vi "WildBugChilGru_V0.189.vi"() -> ()   [LabVIEW 2014]
uses:
  <vilib>/Utility/miscctls.llb/LVPointTypeDef.ctl
  <vilib>/Analysis/NI_AALBase.lvlib
  <vilib>/gmath/NI_Gmath.lvlib
  <vilib>/Analysis/NI_AALPro.lvlib
  <vilib>/Utility/NIReport.llb/NI_report.lvclass
  <vilib>/Utility/NIReport.llb/Append Report Text (str wrap).vi
  <vilib>/Instr/_visa.llb/VISA Configure Serial Port (Instr).vi
  <vilib>/Analysis/3filter.llb/IIR Filter (DBL).vi
  <vilib>/Utility/xml.llb/Read From XML File(string).vi
  <vilib>/Utility/xml.llb/Write to XML File(string).vi
panel:
  in  "Registerkarte 2":T1(tab)
  in  "Gleitender Mittelwert":u8=35
  in  "Differenzenquotient":u8=12
  in  "Polynom":u8=15
  in  "n vom Gas [1/min]":dbl=5000.0
  in  "Zündung [Imp/U]":u8=5
  in  "Übersetzung ermitteln aus":T2(ring)
  in  "Getriebe [1:]":dbl=5.343
  in  "Reifenumfang [m]":dbl=1.222
  in  "Dauer [s]":dbl=5.0
  in  "nKuWe/nRolle":dbl=10.0
  in  "Rolle [Inkr/U]":u16=10
  in  "Rollenumfang [m]":dbl=0.613
  in  "Rollenträgheit [kgm²]":dbl=0.402
  in  "Lufttemperatur [°C]":dbl=20.0
  in  "Luftfeuchtigkeit [%]":dbl=50.0
  in  "Luftdruck [mbar]":dbl=1013.0
  in  "Messung":bool
  in  "Ende":bool
  out "Datenspeicher":T3
  out "COM-Fehlerrate":string="0 / 0,0%"
  in  "Konfiguration:":bool
  in  "Speichern":bool
  in  "Drucken":bool
  out "Pmax":string="0,0 PS"
  out "Ergebnis":string="0,0 PS bei 0 1/min   |   0,0 Nm bei 0 1/min   |   vmax: 2147483647 km/h\nDIN 70020 k =1,000 (20 °C, 50 %, 1013 mbar)\n20.11.2016 20:05 "
  in  "Fahrzeugdaten":string="Hier die Fahrzeugdaten eingeben"
  out "XY-Graph":cluster{dbl[], dbl[]}[](graph)
  out "Untersetzung\nermittelt":bool
  out "Untersetzung":dbl format="%#.2f"
  in  "Start [F1]":bool
  out "Füllstand Lesepuffer":u64(slide) scale=1.0..100.0
  out "Hinterrad\n[km/h]":dbl(knob) scale=0.0..150.0
  out "Welle\n[1/min]":cluster{dbl, dbl}(knob) scale=0.0..12000.0
  out "Lesepuffer":string="\n"
  in  "Serielle Schnittstelle":refnum<visa-resource-name>="COM6"
  out "Untersetzung-Graph":dbl(graph)=2.6802446808510636 caption="Untersetzung"
  # "1. n konstant halten\n2. START\n3. n weiter halten\n4. bei GO: Vollgas\n5. vom Gas gehen"
  # "Go"
  # "Zündung\nRolle"
  # "Untersetzung aus:"
  # "Lesen <> Messen"
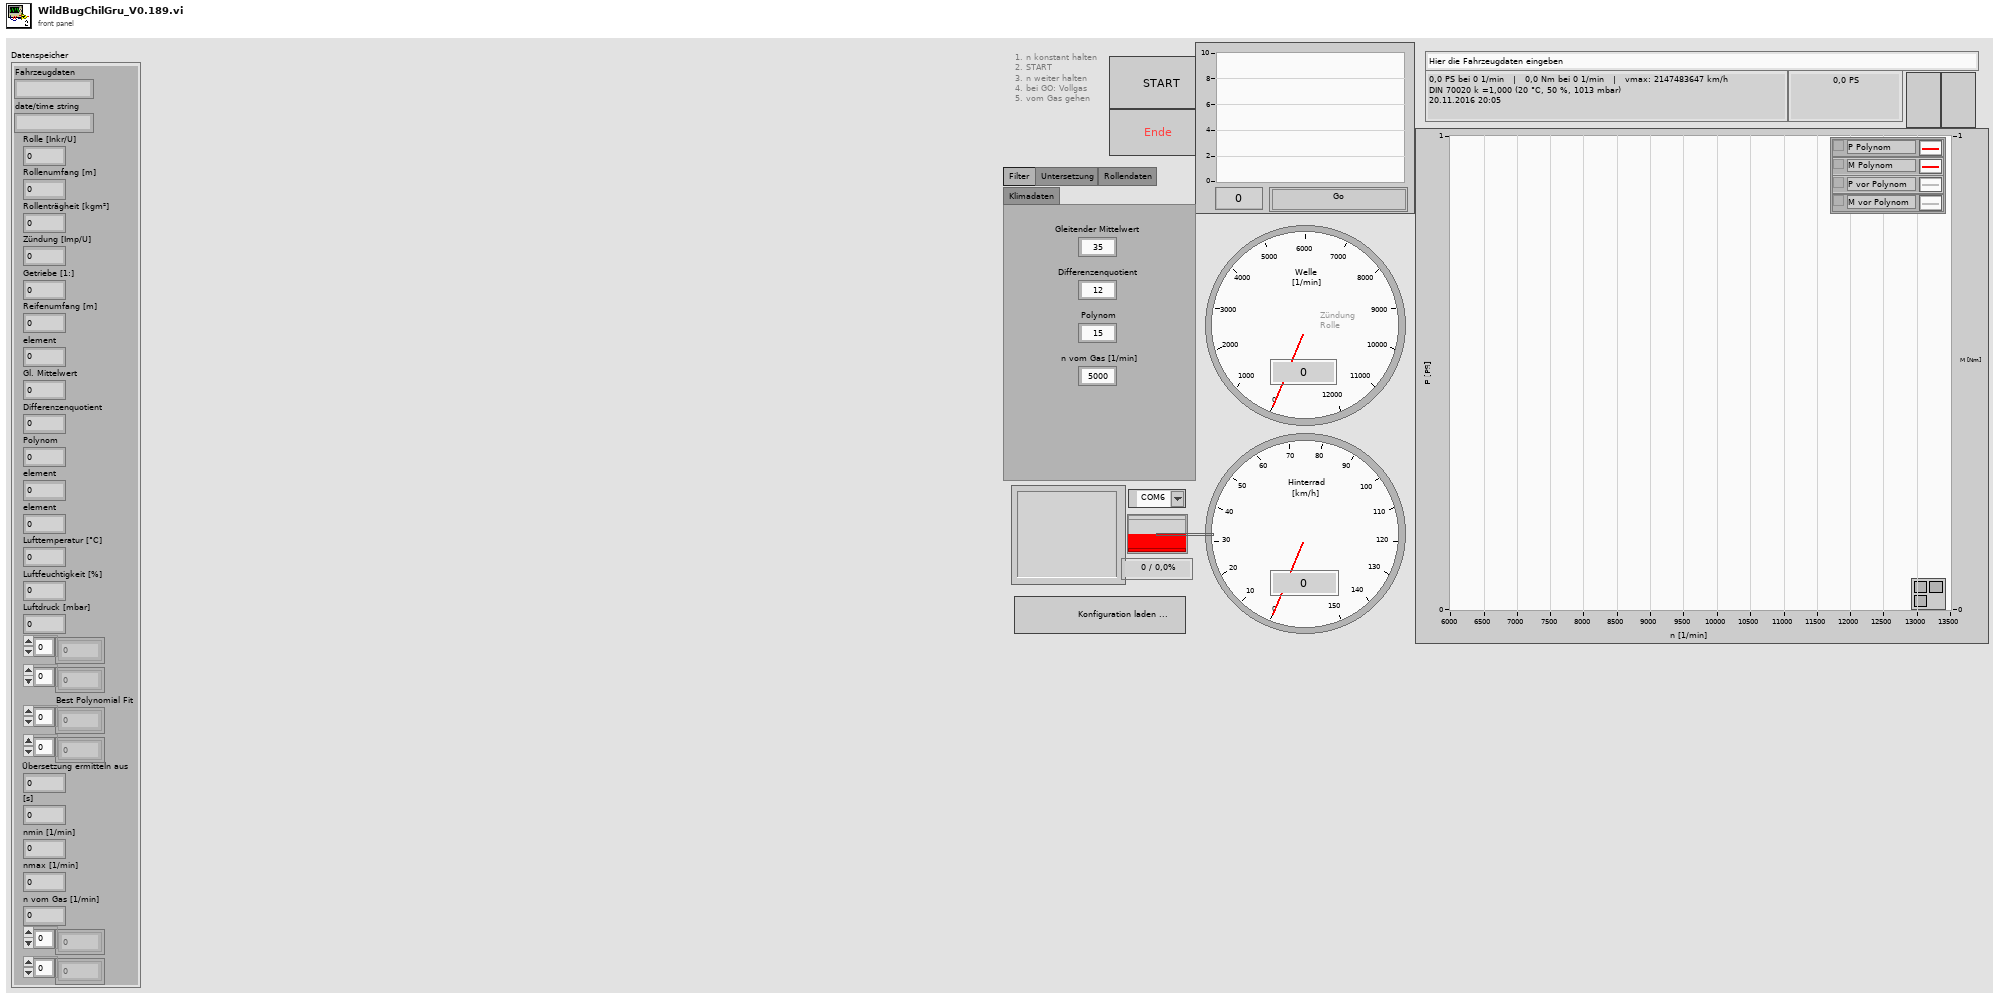
[diagram p1: front panel]
types:
  T1 = enum32{"Filter", "Untersetzung", "Rollendaten", "Klimadaten"}
  T2 = enum8{"Zündsignal", "Getriebe & Reifen", "nKuWe / nRolle"}
  T3 = cluster{"Fahrzeugdaten":string, "date/time string":string, "Rolle [Inkr/U]":u16, "Rollenumfang [m]":dbl, "Rollenträgheit [kgm²]":dbl, "Zündung [Imp/U]":u8, "Getriebe [1:]":dbl, "Reifenumfang [m] ":dbl, "element":dbl, "Gl. Mittelwert":u8, "Differenzenquotient":u8, "Polynom":u8, "element":dbl, "element":dbl, "Lufttemperatur [°C]":dbl, "Luftfeuchtigkeit [%]":dbl, "Luftdruck [mbar]":dbl, dbl[], dbl[], "Best Polynomial Fit":dbl[], dbl[], "Übersetzung ermitteln aus":u8, "[s]":dbl, "nmin [1/min]":dbl, "nmax [1/min]":dbl, "n vom Gas [1/min]":dbl, dbl[], i32[]}
  T4 = enum16{"Kleinste Quadrate", "Kleinestes absolutes Reiduum", "Biquadrat"}
  T5 = enum8{"Enabled", "Disabled", "Disabled and Grayed Out"}
  T6 = cluster{"Fahrzeugdaten":string, "date/time string":string, "Rolle [Inkr/U]":u16, "Rollenumfang [m]":dbl, "Rollenträgheit [kgm²]":dbl, "Zündung [Imp/U]":u8, "Getriebe [1:]":dbl, "Reifenumfang [m] ":dbl, "mean value":dbl, "Gleitender Mittelwert":u8, "Differenzenquotient":u8, "Polynom":u8, dbl, "element":dbl, "Lufttemperatur [°C]":dbl, "Luftfeuchtigkeit [%]":dbl, "Luftdruck [mbar]":dbl, dbl[], dbl[], "Best Polynomial Fit":dbl[], dbl[], "Übersetzung ermitteln aus":enum8{"Zündsignal", "Getriebe & Reifen", "nKuWe / nRolle"}, "Dauer [s]":dbl, dbl, dbl, "n vom Gas [1/min]":dbl, dbl[], i32[]}
  T7 = typedef "LVPointTypeDef.ctl" = cluster{"Horizontal":i16, "Vertical":i16}
  T8 = cluster{string, string, u16, dbl, dbl, u8, dbl, dbl, dbl, u8, u8, u8, dbl, dbl, dbl, dbl, dbl, dbl[], dbl[], dbl[], dbl[], i32, dbl, dbl, dbl, dbl, dbl[], i32[]}
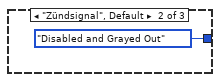
[diagram p2: hidden frame]
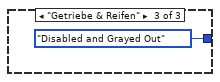
[diagram p3: hidden frame]
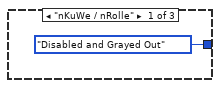
[diagram p4: hidden frame]
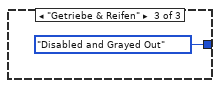
[diagram p5: hidden frame]
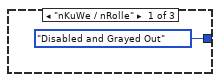
[diagram p6: hidden frame]
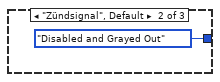
[diagram p7: hidden frame]
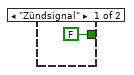
[diagram p10: hidden frame]
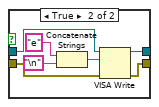
[diagram p12: hidden frame]
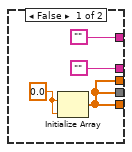
[diagram p14: hidden frame]
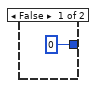
[diagram p15: hidden frame]
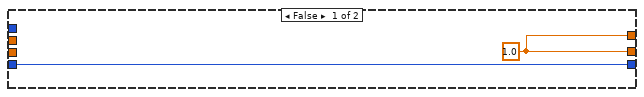
[diagram p17: hidden frame]
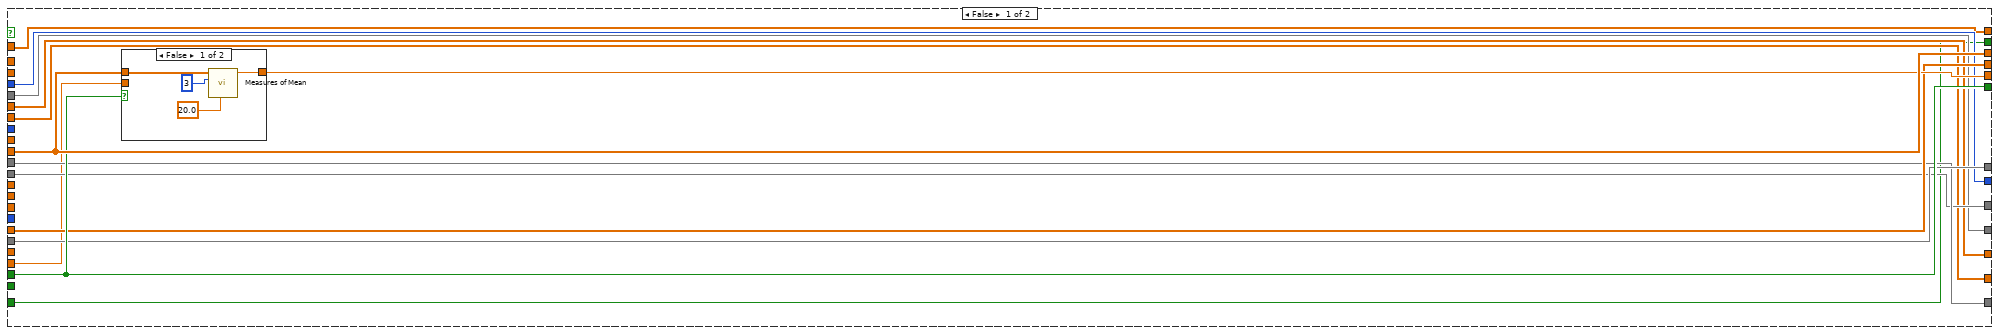
[diagram p18: hidden frame]
diagram:
  n1 = while {
    stop <- w1 stop-if-true
    n2 = event shown="[0] \"Start [F1]\": Wertänderung" {
      selector: _ -> [_ _]
      dyn-events: _ -> [_ _]
      timeout: _ -> [_ _]
      tunnel: [_ TRUE] -> w1
      event "Start [F1]": Value Change {
        n3 = event-data() -> ("NewVal"=w2:bool)  [unwired: 1 in, 5 out]
        n4 = case shown="True" w2 {
          frame False {
          }
          frame True {
            n5 = flat-sequence {
              tunnel: [w132] -> w117
              tunnel: [w131] -> w116
              tunnel: ["Messung"] -> w115
              tunnel: w117 -> [w145]
              tunnel: w116 -> [w144]
              tunnel: [0] -> w114
              tunnel: [1.0 ("element")] -> w113
              tunnel: [FALSE] -> w112
              tunnel: [w157] -> w111
              tunnel: [0] -> w110
              tunnel: [w155] -> w109
              tunnel: [-5] -> w108
              tunnel: [w153] -> w107
              tunnel: [w151] -> w106
              tunnel: [w150] -> w105
              tunnel: [0.0] -> w104
              tunnel: [w145] -> w103
              tunnel: [w144] -> w102
              tunnel: w115 -> [w143]
              tunnel: [w143] -> w101
              tunnel: w114 -> [w182]
              tunnel: [w182] -> w100
              tunnel: w113 -> [w181]
              tunnel: [w181] -> w99
              tunnel: w112 -> [w180]
              tunnel: [w180] -> w98
              tunnel: w111 -> [w179]
              tunnel: [w179] -> w97
              tunnel: w110 -> [w178]
              tunnel: [w178] -> w96
              tunnel: w109 -> [w177]
              tunnel: [w177] -> w95
              tunnel: w108 -> [w176]
              tunnel: [w176] -> w94
              tunnel: w107 -> [w175]
              tunnel: [w175] -> w93
              tunnel: w106 -> [w174]
              tunnel: [w174] -> w92
              tunnel: w105 -> [w173]
              tunnel: [w173] -> w91
              tunnel: w104 -> [w172]
              tunnel: [w172] -> w90
              tunnel: w103 -> [w171]
              tunnel: [w168] -> w89
              tunnel: w102 -> [w170]
              tunnel: [w169] -> w88
              tunnel: [w167] -> w87
              tunnel: w101 -> [w167]
              tunnel: w100 -> [w206]
              tunnel: [w206] -> w86
              tunnel: w99 -> [w205]
              tunnel: [w205] -> w85
              tunnel: w98 -> [w204]
              tunnel: [w204] -> w84
              tunnel: w97 -> [w203]
              tunnel: [w203] -> w83
              tunnel: w96 -> [w202]
              tunnel: [w202] -> w82
              tunnel: w95 -> [w201]
              tunnel: [w201] -> w81
              tunnel: w94 -> [w200]
              tunnel: [w200] -> w80
              tunnel: w93 -> [w199]
              tunnel: [w199] -> w79
              tunnel: w92 -> [w198]
              tunnel: [w198] -> w78
              tunnel: w91 -> [w197]
              tunnel: [w197] -> w77
              tunnel: w90 -> [w196]
              tunnel: [w196] -> w76
              tunnel: w89 -> [w195]
              tunnel: [w195] -> w75
              tunnel: w88 -> [w194]
              tunnel: [w194] -> w74
              tunnel: w87 -> [w192]
              tunnel: [w192] -> w73
              tunnel: w86 -> [w222]
              tunnel: [w222] -> w72
              tunnel: w85 -> [w221]
              tunnel: [w221] -> w71
              tunnel: w84 -> [w220]
              tunnel: [w220] -> w70
              tunnel: w83 -> [w219]
              tunnel: [w219] -> w69
              tunnel: w82 -> [w218]
              tunnel: [w218] -> w68
              tunnel: w81 -> [w217]
              tunnel: [w217] -> w67
              tunnel: w80 -> [w216]
              tunnel: [w216] -> w66
              tunnel: w79 -> [w215]
              tunnel: [w215] -> w65
              tunnel: w78 -> [w214]
              tunnel: [w214] -> w64
              tunnel: w77 -> [w213]
              tunnel: [w213] -> w63
              tunnel: w76 -> [w212]
              tunnel: [w212] -> w62
              tunnel: w75 -> [w211]
              tunnel: [w210] -> w61
              tunnel: w74 -> [w208]
              tunnel: [w209] -> w60
              tunnel: w73 -> [w207]
              tunnel: w72 -> [w298]
              tunnel: w71 -> [w297]
              tunnel: w70 -> [w296]
              tunnel: w69 -> [w295]
              tunnel: w68 -> [w294]
              tunnel: w67 -> [w293]
              tunnel: w66 -> [w292]
              tunnel: w65 -> [w291]
              tunnel: w64 -> [w290]
              tunnel: w63 -> [w289]
              tunnel: w62 -> [w288]
              tunnel: w61 -> [w253]
              tunnel: [w298] -> w59
              tunnel: [w297] -> w58
              tunnel: [w296] -> w57
              tunnel: [w295] -> w56
              tunnel: [w294] -> w55
              tunnel: [w293] -> w54
              tunnel: [w292] -> w53
              tunnel: [w291] -> w52
              tunnel: [w290] -> w51
              tunnel: [w289] -> w50
              tunnel: [w288] -> w49
              tunnel: [w253] -> w48
              tunnel: [w252] -> w47
              tunnel: [w287] -> w46
              tunnel: [w286] -> w45
              tunnel: [w285] -> w44
              tunnel: ["Gleitender Mittelwert"] -> w43
              tunnel: w60 -> [w252]
              tunnel: [w306] -> w9
              tunnel: [w307] -> w10
              tunnel: [w308] -> w11
              tunnel: [w309] -> w12
              tunnel: [w300] -> w7
              tunnel: [w299] -> w8
              tunnel: [w310] -> w13
              tunnel: [w311] -> w14
              tunnel: [w312] -> w16
              tunnel: [w313] -> w18
              tunnel: [w314] -> w19
              tunnel: [w315] -> w20
              tunnel: [w316] -> w37
              tunnel: [w317] -> w39
              tunnel: [w318] -> w40
              tunnel: [w319] -> w41
              tunnel: [w320] -> w42
              tunnel: w59 -> [w320]
              tunnel: w58 -> [w319]
              tunnel: w57 -> [w318]
              tunnel: w56 -> [w317]
              tunnel: w55 -> [w316]
              tunnel: w54 -> [w315]
              tunnel: w53 -> [w314]
              tunnel: w52 -> [w313]
              tunnel: w51 -> [w312]
              tunnel: w50 -> [w311]
              tunnel: w49 -> [w310]
              tunnel: w48 -> [w302]
              tunnel: w47 -> [w301]
              tunnel: w46 -> [w309]
              tunnel: w45 -> [w308]
              tunnel: w44 -> [w307]
              tunnel: w43 -> [w306]
              frame #0 {
                w137 = u16 0 items=["None", "XON/XOFF", "RTS/CTS", "XON/XOFF & RTS/CTS", "DTR/DSR", "XON/XOFF & DTR/DSR"] ("flow control (0:none)")
                w138 = u16 10 items=["1.0"=10, "1.5"=15, "2.0"=20] ("stop bits (10: 1 bit)")
                w130 = FALSE  # Enable Termination Char (T)
                w133 = u32 10000  # timeout (10sec)
                n6 = call-poly "VISA Configure Serial Port"("VISA resource name"="Serielle Schnittstelle", "timeout (10sec)"=w133, "Enable Termination\nChar (T)"=w130, "baud rate (9600)"=u32 250000 ("baudrate (250000)"), "data bits (8)"=u16 8, "parity (0:none)"=enum16{"None", "Odd", "Even", "Mark", "Space"}."None", "stop bits (10: 1 bit)"=w138, "flow control (0:none)"=w137) -> ("VISA resource name out"=w135:refnum<visa-resource-name>, "error out"=w134:errorcluster)  [unwired: 6 in]
                n7 = VISA Clear(VISA resource name=w135, error in (no error)=w134) -> (VISA resource name out=w132:refnum<visa-resource-name>, error out=w131:errorcluster)
              }
              frame #1 {
                w146 = T5."Disabled and Grayed Out" ("Deaktiviert")
                w149 = 0.0  # Graphen löschen
                w152 = 0
                w158 = 0.0
                w150 = ""
                n8 = case shown="True" w143 {
                  frame False {
                  }
                  frame True {
                    n9 = Wait (ms)(milliseconds to wait=u32 2000 ("Zu wartende ms")) -> ()  [unwired: 1 out]
                  }
                }
                n10 = local read "Übersetzung ermitteln aus"() -> (w142:T2)
                n11 = Build Array(w149) -> (w148:dbl[])
                n12 = local write "Pmax"(w150) -> ()
                n13 = property on="Drucken" class="Bool. (strikt)"("DisabledEnum"=w146) -> ()  [unwired: 2 in, 2 out]
                n14 = property on="Übersetzung ermitteln aus" class="Enum (strikt)"("DisabledEnum"=w146) -> ()  [unwired: 2 in, 2 out]
                n15 = property on="Konfiguration:" class="Bool. (strikt)"("DisabledEnum"=w146) -> ()  [unwired: 2 in, 2 out]
                n16 = property on="Ende" class="Bool. (strikt)"("DisabledEnum"=w146) -> ()  [unwired: 2 in, 2 out]
                n17 = property on="Speichern" class="Bool. (strikt)"("DisabledEnum"=w146) -> ()  [unwired: 2 in, 2 out]
                n18 = property on="Untersetzung-Graph" class="SVDiagr (strikt)"("History Data"=w148) -> ()  [unwired: 2 in, 2 out]
                n19 = local write "COM-Fehlerrate"(w150) -> ()
                n20 = local write "Ergebnis"(w150) -> ()
                n21 = case shown="\"Getriebe & Reifen\", Standard" w142 {
                  tunnel: [FALSE TRUE] -> w155
                  frame "Zündsignal" {
                  }
                  frame "Getriebe & Reifen", Default {
                  }
                }
                n22 = Initialize Array(0.0 ("y"), 0) -> (w153:dbl[])
                n23 = Initialize Array(w152, w152) -> (w151:i32[])
                n24 = Initialize Array(w158, w158) -> (w157:dbl[])
              }
              frame #2 {
                n25 = case shown="False" w167 {
                  tunnel: w171 -> [w184 w188]
                  tunnel: w170 -> [w183 w187]
                  tunnel: [w183 w186] -> w169
                  tunnel: [w184 w185] -> w168
                  frame False {
                  }
                  frame True {
                    n26 = Concatenate Strings("e" ("String"), "\n") -> (w191:string)
                    n27 = VISA Write(VISA resource name=w188, write buffer=w191, error in (no error)=w187) -> (VISA resource name out=w185:refnum<visa-resource-name>, error out=w186:errorcluster)  [unwired: 1 out]
                  }
                }
              }
              frame #3 {
                n28 = Wait (ms)(milliseconds to wait=u32 500 ("Zu wartende ms")) -> ()  [unwired: 1 out]
              }
              frame #4 {
                n29 = case shown="True" w207 {
                  tunnel: w211 -> [w224 w247]
                  tunnel: [w224 w246] -> w210
                  tunnel: [w223 w245] -> w209
                  tunnel: w208 -> [w223 w244]
                  frame False {
                  }
                  frame True {
                    n30 = property class="Instr"(reference=w247, error in=w244) -> (reference out=w250:refnum<visa-resource-name>, error out=w249:errorcluster, "Serial Settings:Number of Bytes at Serial Port"=w248:u32)
                    n31 = VISA Read(VISA resource name=w250, byte count=w248, error in (no error)=w249) -> (VISA resource name out=w246:refnum<visa-resource-name>, read buffer=w235:string, error out=w245:errorcluster)  [unwired: 1 out]
                    n32 = Search and Replace String(replace all?=TRUE ("Alle ersetzen? (F)"), input string=w235, search string="." ("Such-String"), replace string="," ("Ersetzungs-String (\"\")")) -> (result string=w234:string)  [unwired: 4 in, 3 out]
                    n33 = String Subset(string=w234, offset (0)=1 ("Offset (0)"), length (rest)=4 ("Länge (Rest)")) -> (substring=w233:string)
                    n34 = String Subset(string=w234, offset (0)=6 ("Offset (0)"), length (rest)=6 ("Länge (Rest)")) -> (substring=w231:string)
                    n35 = String Subset(string=w234, offset (0)=13 ("Offset (0)"), length (rest)=4 ("Länge (Rest)")) -> (substring=w230:string)
                    n36 = Fract/Exp String To Number(string=w233) -> (number=w232:dbl)  [unwired: 3 in, 1 out]
                    n37 = Fract/Exp String To Number(string=w231) -> (number=w227:dbl)  [unwired: 3 in, 1 out]
                    n38 = local write "Lufttemperatur [°C]"(w232) -> ()
                    n39 = Fract/Exp String To Number(string=w230) -> (number=w229:dbl)  [unwired: 3 in, 1 out]
                    n40 = Divide(x=w227, y=100.0 ("x")) -> (x/y=w228:dbl)
                    n41 = local write "Luftdruck [mbar]"(w228) -> ()
                    n42 = local write "Luftfeuchtigkeit [%]"(w229) -> ()
                  }
                }
              }
              frame #5 {
                n43 = Wait (ms)(milliseconds to wait=u32 2000 ("Zu wartende ms")) -> ()  [unwired: 1 out]
                n44 = Add(x="Lufttemperatur [°C]", y=273.15) -> (x+y=w268:dbl)
                n45 = Divide ("M_Welle [Nm]")(x=300.0, y=w268) -> (x/y=w271:dbl)
                n46 = Multiply(x="Luftfeuchtigkeit [%]", y=0.01) -> (x*y=w282:dbl)
                n47 = Divide ("M_Welle [Nm]")(x=w268, y=293.15) -> (x/y=w266:dbl)
                n48 = Multiply(x=w282, y=240800000000.0) -> (x*y=w256:dbl)
                n49 = Power Of X(1:w271, 2:5.0) -> (0:w269:dbl)
                n50 = Multiply(x=w256, y=w269) -> (x*y=w276:dbl)
                n51 = Multiply(x=w271, y=-22.644) -> (x*y=w277:dbl)
                n52 = Power Of X(1:w266, 2:0.5) -> (0:w263:dbl)
                n53 = Exponential(1:w277) -> (0:w275:dbl)
                n54 = Multiply(x=w276, y=w275) -> (x*y=w274:dbl)
                n55 = Subtract "p_Trocken [mbar]"(x="Luftdruck [mbar]", y=w274) -> (x-y=w272:dbl)
                n56 = Divide ("M_Welle [Nm]")(x=1013.0, y=w272) -> (x/y=w264:dbl)
                n57 = Multiply "Korrekturfaktor DIN 70020"(x=w264, y=w263) -> (x*y=w287:dbl)
                n58 = Divide(x="Gleitender Mittelwert", y=2) -> (x/y=w260:dbl)
                n59 = Round Toward -Infinity(1:w260) -> (0:w259:dbl)
                n60 = call <vilib>:"Smoothing Filter Coefficients.vi"("shape"=1, "half-width"=w259, "type"=0) -> ("forward coefficients"=w285:dbl[], "reverse coefficients"=w286:dbl[])  [unwired: 6 in, 1 out]
              }
              frame #6 {
                n61 = Concatenate Strings("m" ("String"), "\n") -> (w305:string)
                n62 = VISA Write(VISA resource name=w302, write buffer=w305, error in (no error)=w301) -> (VISA resource name out=w299:refnum<visa-resource-name>, error out=w300:errorcluster)  [unwired: 1 out]
              }
            }
            n63 = while {
              tunnel: w8 -> [w449]
              tunnel: w7 -> [w448]
              shift-right: [w521] -> _
              shift-left: w14 -> [w465]
              shift-right: [w516] -> _
              shift-left: w13 -> [w520]
              shift-right: [w515] -> _
              shift-left: w13 -> [w519]
              shift-right: [w469] -> _
              shift-left: w13 -> [w518]
              shift-right: [w497] -> _
              shift-left: w42 -> [w517]
              shift-right: [w457] -> w25
              shift-left: w41 -> [_]
              shift-right: [w475] -> w29
              shift-left: w13 -> [w498]
              shift-right: [w508] -> w27
              shift-left: w13 -> [w471]
              shift-right: [w470] -> _
              shift-left: w18 -> [w512]
              shift-right: [w509] -> _
              shift-left: w40 -> [w486]
              shift-right: [w450] -> _
              shift-left: w39 -> [_]
              shift-right: [w456] -> _
              shift-left: w39 -> [_]
              shift-right: [w507] -> w28
              shift-left: w39 -> [w505]
              shift-right: [w506] -> _
              shift-left: w39 -> [w504]
              shift-right: [w492] -> w36
              shift-left: w18 -> [w503]
              shift-right: [w496] -> _
              shift-left: w18 -> [w501]
              shift-right: [w495] -> w32
              shift-left: w18 -> [w502]
              shift-right: [w494] -> w35
              shift-left: w18 -> [w500]
              shift-right: [w493] -> w34
              shift-left: w18 -> [w499]
              tunnel: [w491] -> w38
              shift-right: [w487] -> w33
              shift-left: w37 -> [w489]
              tunnel: [w490] -> w3
              tunnel: ["n vom Gas [1/min]"] -> w31
              tunnel: ["Rollenumfang [m]"] -> w30
              tunnel: ["Rollenumfang [m]"] -> w24
              shift-right: [w482] -> _
              shift-left: w20 -> [w483]
              shift-right: [w476] -> _
              shift-left: w19 -> [w481]
              shift-right: [w477] -> _
              shift-left: w13 -> [w480]
              shift-right: [w478] -> _
              shift-left: w13 -> [w479]
              shift-right: [w474] -> w17
              shift-left: w18 -> [w473]
              shift-right: [w468] -> _
              shift-left: _ -> [w467]
              shift-right: [w472] -> w15
              shift-left: w16 -> [w466]
              tunnel: [w464] -> w4
              tunnel: w12 -> [w457]
              tunnel: w11 -> [w450]
              tunnel: w10 -> [w456]
              tunnel: w9 -> [w455]
              stop <- w491 stop-if-true
              n64 = property class="Instr"(reference=w449, error in=w448) -> (reference out=w460:refnum<visa-resource-name>, error out=w459:errorcluster, "Serial Settings:Number of Bytes at Serial Port"=w462:u32)
              n65 = Greater?(x=w462, y=u32 1 ("min. Bytes")) -> (0:w458:bool)
              n66 = case shown="True" w458 {
                tunnel: w462 -> [_ w523]
                tunnel: [u32 0 ("Bytes at Port") w523] -> w461
                frame False {
                }
                frame True {
                }
              }
              n67 = case shown="1.." w461 {
                selector: w461 -> [_ w769]
                tunnel: [w719 w763] -> w490
                tunnel: [w718 w764] -> w464
                tunnel: [w723 w765] -> w515
                tunnel: [w724 w762] -> w516
                tunnel: w465 -> [w725 w760]
                tunnel: [w725 w758] -> w521
                tunnel: w520 -> [w724 w750]
                tunnel: w519 -> [w723 w749]
                tunnel: [w720 w748] -> w469
                tunnel: w518 -> [w720 w747]
                tunnel: w517 -> [w722 _]
                tunnel: [w722 w730] -> w497
                tunnel: [w721 w736] -> w468
                tunnel: w467 -> [w721 w735]
                tunnel: w460 -> [w718 w727]
                tunnel: w459 -> [w719 w726]
                frame 0, Default {
                  # "No data in from serial port - Nothing to do."
                }
                frame 1.. {
                  # "Hz Drum"
                  n68 = VISA Read(VISA resource name=w727, byte count=w769, error in (no error)=w726) -> (VISA resource name out=w764:refnum<visa-resource-name>, read buffer=w761:string, error out=w763:errorcluster)  [unwired: 1 out]
                  n69 = Concatenate Strings(w760, w761) -> (w732:string)
                  "Lesepuffer" <- w732
                  n70 = Spreadsheet String To Array(delimiter (Tab)="\n" ("regular expression"), format string="%s" ("regular expression"), spreadsheet string=w732, array type (2D Dbl)=string[] [] ("Array 2")) -> (array=w741:string[])
                  n71 = Match Pattern(string=w732, regular expression="[\\n]") -> (before substring=w739:string, after substring=w759:string, offset past match=w773:i32)  [unwired: 1 in, 1 out]
                  n72 = Array Size(array=w741) -> (size(s)=w745:i32)
                  n73 = Match Pattern(string=w739, regular expression="[;]") -> (before substring=w737:string, after substring=w738:string, offset past match=w734:i32)  [unwired: 1 in, 1 out]
                  n74 = Subtract "aktuelle Zeilenanzahl"(x=w745, y=1) -> (x-y=w730:i32)
                  n75 = property on="Füllstand Lesepuffer" class="Schieber (strikt)"() -> ("Scale.Maximum"=w729:dbl)  [unwired: 2 in, 2 out]
                  n76 = Match Pattern(string=w738, regular expression="[;]") -> (before substring=w768:string, after substring=w771:string, offset past match=w756:i32)  [unwired: 1 in, 1 out]
                  n77 = Match Pattern(string=w771, regular expression="[;]") -> (before substring=w767:string, after substring=w766:string, offset past match=w754:i32)  [unwired: 1 in, 1 out]
                  n78 = Greater?(x=w730, y=w729) -> (0:w731:bool)
                  n79 = Greater Or Equal To 0?(x=w734) -> (x >= 0?=w733:bool)
                  n80 = Greater Or Equal To 0?(x=w754) -> (x >= 0?=w753:bool)
                  n81 = Greater Or Equal To 0?(x=w756) -> (x >= 0?=w755:bool)
                  n82 = Greater Or Equal To 0?(x=w773) -> (x >= 0?=w757:bool)
                  n83 = Select(t=w730, s=w731, f=w729) -> (s? t:f=w728:dbl)
                  n84 = property on="Füllstand Lesepuffer" class="Schieber (strikt)"("Scale.Maximum"=w728) -> ()  [unwired: 2 in, 2 out]
                  n85 = Build Array(w757, w755, w733, w753) -> (w752:bool[])
                  n86 = And Array Elements(Boolean array=w752) -> (logical AND=w751:bool)
                  n87 = case shown="True" w751 {
                    tunnel: w768 -> [_ w784]
                    tunnel: w767 -> [_ w789]
                    tunnel: w766 -> [_ w788]
                    tunnel: [w777 w787] -> w765
                    tunnel: [w778 w786] -> w762
                    tunnel: w759 -> [_ w785]
                    tunnel: [w779 w785] -> w758
                    tunnel: w732 -> [w779 _]
                    tunnel: w750 -> [w778 _]
                    tunnel: w749 -> [w777 _]
                    tunnel: [w776 w783] -> w748
                    tunnel: w747 -> [w776 _]
                    tunnel: w737 -> [_ w782]
                    tunnel: [w775 w780] -> w736
                    tunnel: w735 -> [w775 _]
                    frame False {
                    }
                    frame True {
                      # "Cyclecounter"
                      # "Hz ComLevel"
                      # "ComLevel\nLevel 10 =   6Hz \nLevel 5 =   12Hz \nLevel 4 =   15Hz\nLevel 3 =   20Hz\nLevel 2 =   33Hz\nLevel 1 =   62Hz"
                      # "Hz Drum"
                      # "Hz Engine"
                      # "t4m"
                      n88 = Fract/Exp String To Number(string=w782) -> (number=w781:dbl)  [unwired: 3 in, 1 out]
                      n89 = Fract/Exp String To Number(string=w788) -> (number=w787:dbl)  [unwired: 3 in, 1 out]
                      n90 = Fract/Exp String To Number(string=w784) -> (number=w783:dbl)  [unwired: 3 in, 1 out]
                      n91 = To Long Integer(number=w781) -> (32bit integer=w780:i32)
                      n92 = Fract/Exp String To Number(string=w789) -> (number=w786:dbl)  [unwired: 3 in, 1 out]
                    }
                  }
                }
              }
              "Füllstand Lesepuffer" <- w497
              n93 = Not Equal?(x=w467, y=w468) -> (x != y?=w451:bool)
              n94 = case shown="True" w451 {
                tunnel: w481 -> [w527 w538]
                tunnel: [w527 w550] -> w476
                tunnel: w480 -> [w526 w549]
                tunnel: [w526 w535] -> w477
                tunnel: w479 -> [w525 w548]
                tunnel: [w525 w536] -> w478
                tunnel: w468 -> [_ w534]
                tunnel: w466 -> [w524 w533]
                tunnel: [w524 w537] -> w472
                frame False {
                }
                frame True {
                  n95 = Build Array (concatenate)(w533, w534) -> (w537:i32[])
                  n96 = Greater Or Equal To 0?(x=w538) -> (x >= 0?=w539:bool)
                  n97 = case shown="True" w539 {
                    tunnel: [w551 w562] -> w535
                    tunnel: [w551 w563] -> w536
                    tunnel: [w552 w554] -> w550
                    tunnel: w549 -> [_ w556]
                    tunnel: w548 -> [_ w564]
                    tunnel: w534 -> [w552 w553]
                    tunnel: w538 -> [_ w554]
                    frame False {
                      w551 = 1.0
                    }
                    frame True {
                      w560 = 65536.0
                      n98 = Add(x=w554, y=w556) -> (x+y=w555:dbl)
                      n99 = Divide(x=w555, y=w560) -> (x/y=w565:dbl)
                      n100 = Increment(x=w564) -> (x+1=w563:dbl)
                      n101 = Round Toward -Infinity(1:w565) -> (0:w561:dbl)
                      n102 = Multiply(x=w561, y=w560) -> (x*y=w559:dbl)
                      n103 = Add(x=w559, y=w553) -> (x+y=w558:dbl)
                      n104 = Increment(x=w558) -> (x+1=w557:dbl)
                      n105 = Subtract(x=w557, y=w554) -> (x-y=w562:dbl)
                    }
                  }
                  n106 = Subtract(x=w535, y=w536) -> (x-y=w530:dbl)
                  n107 = Decrement(x=w530) -> (x-1=w529:dbl)
                  n108 = Max & Min(x=0, y=w529) -> (max(x,y)=w528:dbl)  [unwired: 1 out]
                  n109 = Divide(x=w528, y=w535) -> (x/y=w542:dbl)
                  n110 = Greater Than 0?(x=w528) -> (x > 0?=w532:bool)
                  n111 = Select(t=u32 16711680, s=w532, f=u32 0) -> (s? t:f=w543:u32)
                  n112 = Multiply(x=w542, y=100.0) -> (x*y=w540:dbl)
                  n113 = property on="COM-Fehlerrate" class="Str"("Text.TextColor"=w543) -> ()  [unwired: 2 in, 2 out]
                  n114 = Format Into String(format string="%d / %.1f%%" ("Format-String"), w528, w540) -> (resulting string=→"COM-Fehlerrate":string)  [unwired: 2 in, 1 out]
                }
              }
              n115 = case "Case-Struktur" shown="True" w451 {
                tunnel: w516 -> [w699 w710]
                tunnel: w515 -> [w698 w709]
                tunnel: [w699 w708] -> w514
                tunnel: [w698 w707] -> w513
                tunnel: w469 -> [_ w701]
                tunnel: w498 -> [w697 _]
                tunnel: [w697 w700] -> w475
                tunnel: w471 -> [_ w706]
                tunnel: "Rollenumfang [m]" -> [_ w705]
                frame False {
                }
                frame True {
                  w717 = 60.0 ("y")
                  n116 = Reciprocal "Abtastzeit [s]"(x=w701) -> (1/x=w700:dbl)
                  n117 = Divide "R [1/s]"(x=w709, y="Rolle [Inkr/U]") -> (x/y=w716:dbl)
                  n118 = Multiply "nR [1/min]"(x=w717, y=w716) -> (x*y=w707:dbl)
                  n119 = Divide(x=w710, y="Zündung [Imp/U]") -> (x/y=w713:dbl)
                  n120 = Multiply "nZ gemessen [1/min]"(x=w713, y=w717) -> (x*y=w708:dbl)
                  n121 = Multiply "nZ berechnet [1/min]"(x=w707, y=w706) -> (x*y=w715:dbl)
                  n122 = Multiply "[m/min]"(x=w707, y=w705) -> (x*y=w711:dbl)
                  n123 = Multiply "[km/h]"(x=w711, y=0.06) -> (x*y=→"Hinterrad\n[km/h]":dbl)
                  n124 = Bundle(w708, w715) -> (→"Welle\n[1/min]":cluster{dbl, dbl})  [unwired: 1 in]
                }
              }
              n125 = local read "Übersetzung ermitteln aus"() -> (w452:T2)
              n126 = case shown="True" w451 {
                tunnel: w514 -> [_ w634]
                tunnel: w513 -> [_ w633]
                tunnel: "Rollenumfang [m]" -> [_ w637]
                tunnel: [w577 w603] -> w508
                tunnel: w471 -> [w566 w603]
                tunnel: w452 -> [_ w642]
                tunnel: w486 -> [w578 w641]
                tunnel: w512 -> [w579 w640]
                tunnel: [w578 w594] -> w509
                tunnel: [w579 w639] -> w470
                tunnel: w450 -> [_ w636]
                tunnel: w456 -> [_ w635]
                tunnel: [w576 w589] -> w507
                tunnel: [w575 w587] -> w506
                tunnel: w505 -> [w576 w632]
                tunnel: w504 -> [w575 _]
                tunnel: w455 -> [_ w585]
                tunnel: [w574 w609] -> w492
                tunnel: w503 -> [w574 _]
                tunnel: [w573 w624] -> w496
                tunnel: w501 -> [w573 _]
                tunnel: w498 -> [_ w622]
                tunnel: [w572 w610] -> w495
                tunnel: w502 -> [w572 _]
                tunnel: [w571 w626] -> w494
                tunnel: w500 -> [w571 _]
                tunnel: [w570 w625] -> w493
                tunnel: w499 -> [w570 _]
                tunnel: w457 -> [_ w614]
                tunnel: w489 -> [w569 w608]
                tunnel: "n vom Gas [1/min]" -> [_ w596]
                tunnel: [w569 w607] -> w487
                tunnel: w486 -> [_ w606]
                tunnel: w483 -> [w568 w602]
                tunnel: [w568 w601] -> w482
                tunnel: w475 -> [_ w600]
                tunnel: [w567 w599] -> w474
                tunnel: w473 -> [w567 w598]
                frame False {
                  n127 = case shown="False" w578 {
                    tunnel: w579 -> [w583 _]
                    tunnel: [w582 w584] -> w577
                    tunnel: w566 -> [_ w584]
                    frame False {
                      n128 = call <vilib>:"Measures of Mean.vi"("percent (trim)"=20.0, "type"=3, "x array"=w583) -> ("mean value"=w582:dbl)  [unwired: 7 in, 1 out]
                    }
                    frame True {
                    }
                  }
                }
                frame True {
                  w617 = 0.00135962  # [W] in [PS]
                  w628 = 0.10471975511965978  # 2*Pi/60
                  n129 = Build Array (concatenate) "akt. dT in Array einfügen"(w598, w600) -> (w599:dbl[])
                  n130 = case shown="\"Getriebe & Reifen\"" w642 {
                    tunnel: w634 -> [_ _ w696]
                    tunnel: w633 -> [_ _ w695]
                    tunnel: [w691 "nKuWe/nRolle" w694] -> w638
                    tunnel: w637 -> [w692 _ _]
                    frame "Getriebe & Reifen" {
                      n131 = Divide(x=w692, y="Reifenumfang [m]") -> (x/y=w690:dbl)
                      n132 = Multiply(x=w690, y="Getriebe [1:]") -> (x*y=w691:dbl)
                    }
                    frame "nKuWe / nRolle" {
                    }
                    frame "Zündsignal" {
                      n133 = Divide(x=w696, y=w695) -> (x/y=w694:dbl)
                    }
                  }
                  n134 = Build Array (concatenate) "akt. Rollendrehzahl\nin Array einfügen"(w632, w633) -> (w589:dbl[])
                  n135 = Index Array(array=w589, index=1 ("Index")) -> (element=w592:dbl)
                  n136 = Initialize Array(w592, w585) -> (w591:dbl[])
                  n137 = Insert Into Array(array=w589, index=0 ("Index"), new element=w591) -> (w588:dbl[])
                  n138 = call-poly <vilib>:"IIR Filter.vi"("Forward Coefficients"=w635, "Reverse Coefficients"=w636, "X"=w588) -> ("Filtered X"=w586:dbl[])  [unwired: 1 in, 1 out]
                  n139 = Array Subset(array=w586, index=w585) -> (w587:dbl[])  [unwired: 1 in]
                  n140 = Multiply(x=2.0, y=w622) -> (x*y=w621:dbl)
                  n141 = case shown="False" w641 {
                    selector: w641 -> [_ w687]
                    tunnel: w638 -> [w682 _]
                    tunnel: w640 -> [w684 w686]
                    tunnel: [w679 w687] -> w631
                    tunnel: [w683 w686] -> w639
                    tunnel: w602 -> [w680 w685]
                    tunnel: [w679 w685] -> w601
                    frame False {
                      n142 = Build Array (concatenate)(w684, w682) -> (w683:dbl[])
                      n143 = call "Verstrichene Zeit"("Time Target (s)"="Dauer [s]", "Reset"=w680) -> ("Time has Elapsed"=w679:bool)  [unwired: 10 in, 7 out]
                      "Untersetzung-Graph" <- w682
                    }
                    frame True {
                    }
                  }
                  n144 = Array Size "Array-Größe"(array=w587) -> (size(s)=w629:i32)
                  n145 = Square(x=w603) -> (x^2=w627:dbl)
                  n146 = Multiply(x=w587, y=w603) -> (x*y=w609:dbl[])
                  n147 = Divide(x="Rollenträgheit [kgm²]", y=w627) -> (x/y=w615:dbl)
                  n148 = Greater?(x=w629, y=w585) -> (0:w630:bool)
                  n149 = Multiply(x=w609, y=w628) -> (x*y=w624:dbl[])
                  n150 = Multiply(x=w615, y=w614) -> (x*y=w613:dbl)
                  n151 = And(x=w631, y=w630) -> (x .and. y?=w594:bool)
                  n152 = Array Size "Array-Größe"(array=w624) -> (size(s)=w612:i32)
                  n153 = Decrement(x=w612) -> (x-1=w611:i32)
                  n154 = Select(t=w596, s=w594, f=1000000.0) -> (s? t:f=w597:dbl)
                  n155 = Initialize Array(0.0 ("y"), 0) -> (w618:dbl[])
                  n156 = for {
                    N: w612 -> [_]
                    tunnel: "Differenzenquotient" -> [w654]
                    tunnel: w624 -> [w662]
                    tunnel: w611 -> [w653]
                    tunnel: w621 -> [w663]
                    shift-right: [w659] -> w610
                    shift-left: w618 -> [w660]
                    tunnel: w609 -> [w657] mode=indexing
                    tunnel: w608 -> [w645]
                    tunnel: w597 -> [w656]
                    tunnel: [w646] -> w607
                    tunnel: w606 -> [w643]
                    i -> [w647]
                    stop <- w644 stop-if-true
                    n157 = Subtract(x=w653, y=w654) -> (x-y=w655:i32)
                    n158 = Add(x=w647, y=w654) -> (x+y=w670:i32)
                    n159 = Subtract(x=w647, y=w654) -> (x-y=w676:i32)
                    n160 = Greater Or Equal?(x=w647, y=w654) -> (x >= y?=w650:bool)
                    n161 = Greater?(x=w657, y=w656) -> (0:w658:bool)
                    n162 = Max & Min(x=w653, y=w670) -> (min(x,y)=w671:i32)  [unwired: 1 out]
                    n163 = Max & Min(x=w676, y=0) -> (max(x,y)=w674:i32)  [unwired: 1 out]
                    n164 = Less Or Equal?(x=w647, y=w655) -> (x <= y?=w651:bool)
                    n165 = Subtract(x=w671, y=w647) -> (x-y=w672:i32)
                    n166 = Subtract(x=w647, y=w674) -> (x-y=w673:i32)
                    n167 = Max & Min(x=w673, y=w672) -> (min(x,y)=w664:i32)  [unwired: 1 out]
                    n168 = Multiply(x=w664, y=w663) -> (x*y=w661:dbl)
                    n169 = Add(x=w647, y=w664) -> (x+y=w669:i32)
                    n170 = Subtract(x=w647, y=w664) -> (x-y=w668:i32)
                    n171 = Index Array(array=w662, index=w669) -> (element=w666:dbl)
                    n172 = Index Array(array=w662, index=w668) -> (element=w667:dbl)
                    n173 = Subtract(x=w666, y=w667) -> (x-y=w665:dbl)
                    n174 = Divide(x=w665, y=w661) -> (x/y=w652:dbl)
                    n175 = Less Or Equal To 0?(x=w645) -> (x <= 0?=w648:bool)
                    n176 = Less Than 0?(x=w652) -> (x < 0?=w649:bool)
                    n177 = Build Array (concatenate)(w660, w652) -> (w659:dbl[])
                    n178 = Compound Arithmetic op=AND(w649, w658, w648, w650, w651, w643) -> (w644:bool)
                    n179 = case shown="True" w644 {
                      tunnel: w647 -> [_ w678]
                      tunnel: [w677 w678] -> w646
                      tunnel: w645 -> [w677 _]
                      frame False {
                      }
                      frame True {
                      }
                    }
                  }
                  n180 = Multiply(x=w610, y=w613) -> (x*y=w626:dbl[])
                  n181 = Multiply(x=w624, y=w626) -> (x*y=w616:dbl[])
                  n182 = Multiply(x=w617, y=w616) -> (x*y=w625:dbl[])
                }
              }
              "Untersetzung\nermittelt" <- w509
              n183 = local read "Start [F1]"() -> (w454:bool)
              n184 = Not(x=w454) -> (.not. x?=w453:bool)
              n185 = Greater Than 0?(x=w487) -> (x > 0?=w488:bool)
              n186 = Select(t=w508, s=w509, f=0.0) -> (s? t:f=→"Untersetzung":dbl)
              n187 = Or(x=w488, y=w453) -> (x .or. y?=w491:bool)
            }
            n188 = VISA Clear(VISA resource name=w4, error in (no error)=w3) -> (VISA resource name out=w5:refnum<visa-resource-name>, error out=w6:errorcluster)
            n189 = VISA Close(VISA resource name=w5, error in (no error)=w6) -> ()  [unwired: 1 out]
            n190 = case shown="True" w38 {
              tunnel: w36 -> [_ w424]
              tunnel: w35 -> [_ w429]
              tunnel: w34 -> [_ w428]
              tunnel: w33 -> [_ w400]
              tunnel: w32 -> [_ w425]
              tunnel: w31 -> [_ w423]
              tunnel: w30 -> [_ w417]
              tunnel: w25 -> [_ w403]
              tunnel: ["" w402] -> w26
              tunnel: w27 -> [_ w401]
              tunnel: ["" w399] -> _
              tunnel: [w363 w376] -> w23
              tunnel: [w363 w375] -> w22
              tunnel: [w363 w374] -> w21
              frame False {
                w364 = 0.0
                n191 = Initialize Array(w364, w364) -> (w363:dbl[])
              }
              frame True {
                w388 = 735.498  # PS in W
                w394 = 0.10471975511965978  # w = (2 * Pi / 60) * n
                w398 = 0
                n192 = Array Subset "P"(array=w428, length=w400) -> (w420:dbl[])  [unwired: 1 in]
                n193 = Array Subset "M"(array=w429, length=w400) -> (w421:dbl[])  [unwired: 1 in]
                n194 = Array Subset "alpha"(array=w425, length=w400) -> (w426:dbl[])  [unwired: 1 in]
                n195 = Array Subset "n"(array=w424, length=w400) -> (w422:dbl[])  [unwired: 1 in]
                n196 = property on="Pmax" class="Str"("Text.FontSize"=48) -> ()  [unwired: 2 in, 2 out]
                n197 = property on="Ergebnis" class="Str"("Text.FontSize"=18) -> ()  [unwired: 2 in, 2 out]
                n198 = Array Size(array=w426) -> (size(s)=w427:i32)
                n199 = for {
                  N: w427 -> [w447]
                  tunnel: w425 -> [w444]
                  tunnel: w424 -> [w441]
                  tunnel: w423 -> [w438]
                  tunnel: [w436] -> w396
                  i -> [w442]
                  stop <- w437 stop-if-true
                  n200 = Decrement(x=w447) -> (x-1=w446:i32)
                  n201 = Subtract(x=w446, y=w442) -> (x-y=w436:i32)
                  n202 = Index Array(array=w444, index=w436) -> (element=w445:dbl)
                  n203 = Index Array(array=w441, index=w436) -> (element=w440:dbl)
                  n204 = Less?(x=w440, y=w438) -> (x < y?=w439:bool)
                  n205 = Less Or Equal To 0?(x=w445) -> (x <= 0?=w443:bool)
                  n206 = And(x=w443, y=w439) -> (x .and. y?=w437:bool)
                }
                n207 = Increment(x=w396) -> (x+1=w395:i32)
                n208 = Array Subset "P"(array=w420, index=w395) -> (w397:dbl[])  [unwired: 1 in]
                n209 = Array Subset "M"(array=w421, index=w395) -> (w393:dbl[])  [unwired: 1 in]
                n210 = Array Subset "n"(array=w422, index=w395) -> (w376:dbl[])  [unwired: 1 in]
                n211 = local write "Polynom"("Polynom") -> ()
                n212 = Array Max & Min "nmax [1/min]"(array=w376) -> (max value=w419:dbl)  [unwired: 3 out]
                n213 = Bundle(w376, w397) -> (w380:cluster{dbl[], dbl[]})  [unwired: 1 in]
                n214 = Bundle(w376, w393) -> (w381:cluster{dbl[], dbl[]})  [unwired: 1 in]
                n215 = Multiply(x=w376, y=w394) -> (x*y=w390:dbl[])
                n216 = Array Size(array=w376) -> (size(s)=w373:i32)
                n217 = call <vilib>:"General Polynomial Fit.vi"("Y"=w393, "polynomial order"="Polynom", "X"=w376, "method"=T4."Biquadrat" ("Methode"), "algorithm"=3) -> ("Best Polynomial Fit"=w375:dbl[])  [unwired: 7 in, 3 out]
                n218 = Bundle(w376, "Best Polynomial Fit"=w375) -> (w382:cluster{dbl[], "Best Polynomial Fit":dbl[]})  [unwired: 1 in]
                n219 = Multiply(x=w375, y=w390) -> (x*y=w389:dbl[])
                n220 = Multiply(x=w373, y=0.1) -> (x*y=w367:dbl)
                n221 = Multiply(x=w373, y=0.8) -> (x*y=w384:dbl)
                n222 = Array Subset "MPoly ohne die ersten\nund letzten paar %"(array=w375, index=w367, length=w384) -> (w378:dbl[])
                n223 = Array Subset "n ohne die ersten \nund letzten paar %"(array=w376, index=w367, length=w384) -> ()  [unwired: 1 out]
                n224 = Divide(x=w419, y=w401) -> (x/y=w418:dbl)
                n225 = Divide(x=w389, y=w388) -> (x/y=w374:dbl[])
                n226 = Array Subset "PPoly ohne die ersten\nund letzten paar %"(array=w374, index=w367, length=w384) -> (w379:dbl[])
                n227 = Bundle(w376, w374) -> (w383:cluster{dbl[], dbl[]})  [unwired: 1 in]
                n228 = Compound Arithmetic op=MULTIPLY "vmax"(w418, w417, 0.06) -> (w409:dbl)
                n229 = Array Max & Min "Mmax"(array=w378) -> (max value=w386:dbl, max index (indices)=w369:i32)  [unwired: 2 out]
                n230 = Add(x=w367, y=w369) -> (x+y=w368:dbl)
                n231 = Multiply(x=w386, y=1.8) -> (x*y=w430:dbl)
                n232 = Index Array "n(Mmax)"(array=w376, index=w368) -> (element=w410:dbl)
                n233 = Array Max & Min "Pmax"(array=w379) -> (max value=w387:dbl, max index (indices)=w371:i32)  [unwired: 2 out]
                n234 = Build Array(w383, w382, w380, w381) -> (→"XY-Graph":cluster{dbl[], "Best Polynomial Fit":dbl[]}[])
                n235 = Add(x=w367, y=w371) -> (x+y=w370:dbl)
                n236 = local read "Luftfeuchtigkeit [%]"() -> (w413:dbl)
                n237 = Multiply(x=w387, y=1.2) -> (x*y=w431:dbl)
                n238 = local read "Lufttemperatur [°C]"() -> (w412:dbl)
                n239 = local read "Luftdruck [mbar]"() -> (w414:dbl)
                n240 = property on="XY-Graph" class="XYGraph (strikt)"("ActYScl"=1, "YScale.Maximum"=w430, "YScale.Minimum"=w398) -> ()  [unwired: 2 in, 2 out]
                n241 = property on="XY-Graph" class="XYGraph (strikt)"("ActYScl"=w398, "YScale.Maximum"=w431, "YScale.Minimum"=w398) -> ()  [unwired: 2 in, 2 out]
                n242 = Index Array "n(Pmax)"(array=w376, index=w370) -> (element=w415:dbl)
                n243 = Format Into String(format string="%.1f PS" ("Format-String"), w387) -> (resulting string=→"Pmax":string)  [unwired: 2 in, 1 out]
                n244 = Format Date/Time String(time format string (%c)="%x %H:%M ") -> (date/time string=w402:string)  [unwired: 2 in]
                n245 = Format Into String(format string="%.1f PS bei %d 1/min   |   %.1f Nm bei %d 1/min   |   vmax: %d km/h\\nDIN 70020 k =%.3f (%d \\B0C, %d %%, %d mbar)\\n%s" ("Format-String"), w387, w415, w386, w410, w409, w403, w412, w413, w414, w402) -> (resulting string=w399:string)  [unwired: 2 in, 1 out]
                "Ergebnis" <- w399
              }
            }
            n246 = flat-sequence {
              tunnel: w15 -> [w324]
              tunnel: w17 -> [w325]
              tunnel: w21 -> [w326]
              tunnel: w22 -> [w327]
              tunnel: w23 -> [w328]
              tunnel: w24 -> [w329]
              tunnel: w25 -> [w330]
              tunnel: w26 -> [w331]
              tunnel: w27 -> [w332]
              tunnel: w28 -> [w333]
              tunnel: w29 -> [w334]
              tunnel: [w334] -> w128
              tunnel: [w333] -> w127
              tunnel: [w332] -> w126
              tunnel: [w331] -> w125
              tunnel: [w330] -> w124
              tunnel: [w329] -> w123
              tunnel: [w328] -> w122
              tunnel: [w327] -> w121
              tunnel: [w326] -> w120
              tunnel: [w325] -> w119
              tunnel: [w324] -> w118
              tunnel: w128 -> [w362]
              tunnel: w127 -> [w361]
              tunnel: w126 -> [w360]
              tunnel: w125 -> [w359]
              tunnel: w124 -> [w358]
              tunnel: w123 -> [w357]
              tunnel: w122 -> [w356]
              tunnel: w121 -> [w355]
              tunnel: w120 -> [w354]
              tunnel: w119 -> [w353]
              tunnel: w118 -> [w352]
              frame #0 {
                w322 = FALSE ("Start [F1]")
                w323 = 0  # Aktivieren
                n247 = property on="XY-Graph" class="XYGraph (strikt)"("YScale.ScaleFit"=u8 1 ("X-Achse.Achsenanpassung")) -> ()  [unwired: 2 in, 2 out]
                n248 = property on="Speichern" class="Bool. (strikt)"("DisabledEnum"=w323) -> ()  [unwired: 2 in, 2 out]
                n249 = property on="Übersetzung ermitteln aus" class="Enum (strikt)"("DisabledEnum"=w323) -> ()  [unwired: 2 in, 2 out]
                n250 = property on="Konfiguration:" class="Bool. (strikt)"("DisabledEnum"=w323) -> ()  [unwired: 2 in, 2 out]
                n251 = property on="Ende" class="Bool. (strikt)"("DisabledEnum"=w323) -> ()  [unwired: 2 in, 2 out]
                n252 = property on="Drucken" class="Bool. (strikt)"("DisabledEnum"=w323) -> ()  [unwired: 2 in, 2 out]
                n253 = local write "Untersetzung\nermittelt"(w322) -> ()
                n254 = local write "Start [F1]"(w322) -> ()
              }
              frame #1 {
                w336 = 0.0
                n255 = local read "Übersetzung ermitteln aus"() -> (w339:T2)
                n256 = local read "Rollenträgheit [kgm²]"() -> (w349:dbl)
                n257 = local read "Luftfeuchtigkeit [%]"() -> (w341:dbl)
                n258 = local read "Lufttemperatur [°C]"() -> (w342:dbl)
                n259 = local read "Differenzenquotient"() -> (w344:u8)
                n260 = local read "Reifenumfang [m]"() -> (w346:dbl)
                n261 = local read "n vom Gas [1/min]"() -> (w337:dbl)
                n262 = local read "Zündung [Imp/U]"() -> (w348:u8)
                n263 = local read "Luftdruck [mbar]"() -> (w340:dbl)
                n264 = local read "Gleitender Mittelwert"() -> (w345:u8)
                n265 = local read "Rolle [Inkr/U]"() -> (w350:u16)
                n266 = local read "Getriebe [1:]"() -> (w347:dbl)
                n267 = local read "Polynom"() -> (w343:u8)
                n268 = local read "Dauer [s]"() -> (w338:dbl)
                n269 = Bundle("Fahrzeugdaten"="Fahrzeugdaten", "date/time string"=w359, "Rolle [Inkr/U]"=w350, "Rollenumfang [m]"=w357, "Rollenträgheit [kgm²]"=w349, "Zündung [Imp/U]"=w348, "Getriebe [1:]"=w347, "Reifenumfang [m]"=w346, "mean value"=w360, "Gleitender Mittelwert"=w345, "Differenzenquotient"=w344, "Polynom"=w343, w362, "element"=w358, "Lufttemperatur [°C]"=w342, "Luftfeuchtigkeit [%]"=w341, "Luftdruck [mbar]"=w340, w361, w356, "Best Polynomial Fit"=w355, w354, "Übersetzung ermitteln aus"=w339, "Dauer [s]"=w338, w336, w336, "n vom Gas [1/min]"=w337, w353, w352) -> (→"Datenspeicher":T6)  [unwired: 1 in]
              }
            }
          }
        }
      }
      event "Ende": Value Change {
        n270 = event-data() -> ()  [unwired: 1 in, 6 out]
      }
    }
  }
  n271 = flat-sequence {
    frame #0 {
      w807 = 0
      w803 = u8 0
      w801 = 0.0
      w805 = 0.0
      w800 = ""
      w810 = 2  # Deaktivieren
      w812 = 0.0  # Graphen löschen
      n272 = property on="Füllstand Lesepuffer" class="Schieber (strikt)"("Scale.Maximum"=100) -> ()  [unwired: 2 in, 2 out]
      n273 = Initialize Array(w801, w801) -> (w806:dbl[])
      n274 = Initialize Array(w807, w807) -> (w808:i32[])
      n275 = local read "Serielle Schnittstelle"() -> (w798:refnum<visa-resource-name>)
      n276 = property on="Frontpanel-Position" class="Bereich"("Origin"=T7 {"Horizontal"=8, "Vertical"=6}) -> ()  [unwired: 2 in, 2 out]
      n277 = Bundle(w800, w800, u16 0, w805, w805, w803, w805, w805, w805, w803, w803, w803, w805, w805, w805, w805, w805, w806, w806, w806, w806, 0, w805, w805, w805, w805, w806, w808) -> (w799:T8)  [unwired: 1 in]
      n278 = property on="Drucken" class="Bool. (strikt)"("DisabledEnum"=w810) -> ()  [unwired: 2 in, 2 out]
      n279 = property on="Speichern" class="Bool. (strikt)"("DisabledEnum"=w810) -> ()  [unwired: 2 in, 2 out]
      n280 = local write "Datenspeicher"(w799) -> ()
      n281 = VISA Clear(VISA resource name=w798) -> (VISA resource name out=w797:refnum<visa-resource-name>, error out=w796:errorcluster)  [unwired: 1 in]
      n282 = Build Array(w812) -> (w811:dbl[])
      n283 = VISA Close(VISA resource name=w797, error in (no error)=w796) -> (error out=w795:errorcluster)
      n284 = case shown="\"Getriebe & Reifen\"" "Übersetzung ermitteln aus" {
        tunnel: [T5."Disabled and Grayed Out" ("Deaktiviert") T5."Disabled and Grayed Out" ("Deaktiviert") T5."Enabled" ("Deaktiviert")] -> w794
        frame "nKuWe / nRolle" {
        }
        frame "Zündsignal", Default {
        }
        frame "Getriebe & Reifen" {
        }
      }
      n285 = case shown="\"Zündsignal\", Standard" "Übersetzung ermitteln aus" {
        tunnel: [T5."Disabled and Grayed Out" ("Deaktiviert") T5."Enabled" ("Deaktiviert") T5."Disabled and Grayed Out" ("Deaktiviert")] -> w793
        frame "nKuWe / nRolle" {
        }
        frame "Zündsignal", Default {
        }
        frame "Getriebe & Reifen" {
        }
      }
      n286 = case shown="\"nKuWe / nRolle\"" "Übersetzung ermitteln aus" {
        tunnel: [T5."Enabled" ("Deaktiviert") T5."Disabled and Grayed Out" ("Deaktiviert") T5."Disabled and Grayed Out" ("Deaktiviert")] -> w792
        frame "nKuWe / nRolle" {
        }
        frame "Zündsignal", Default {
        }
        frame "Getriebe & Reifen" {
        }
      }
      n287 = property on="Untersetzung-Graph" class="SVDiagr (strikt)"("History Data"=w811) -> ()  [unwired: 2 in, 2 out]
      n288 = case shown="Fehler" w795 {
        frame No Error {
        }
        frame Error {
          n289 = property on="Start [F1]" class="Bool. (strikt)"("DisabledEnum"=T5."Disabled and Grayed Out" ("Deaktiviert")) -> ()  [unwired: 2 in, 2 out]
        }
      }
      n290 = property on="Getriebe [1:]" class="DigWert (strikt)"("DisabledEnum"=w794) -> ()  [unwired: 2 in, 2 out]
      n291 = property on="Reifenumfang [m]" class="DigWert (strikt)"("DisabledEnum"=w794) -> ()  [unwired: 2 in, 2 out]
      n292 = property on="Zündung [Imp/U]" class="DigWert (strikt)"("DisabledEnum"=w793) -> ()  [unwired: 2 in, 2 out]
      n293 = property on="nKuWe/nRolle" class="DigWert (strikt)"("DisabledEnum"=w792) -> ()  [unwired: 2 in, 2 out]
    }
  }
  n294 = while {
    stop <- w824 stop-if-true
    n295 = event shown="[0] \"Konfiguration:\": Wertänderung" {
      selector: _ -> [_ _ _ _ _ _ _]
      dyn-events: _ -> [_ _ _ _ _ _ _]
      timeout: _ -> [_ _ _ _ _ _ _]
      tunnel: [_ _ _ TRUE _ _ _] -> w824
      event "Konfiguration:": Value Change {
        n296 = event-data() -> ("OldVal"=w825:bool)  [unwired: 1 in, 5 out]
        n297 = flat-sequence {
          tunnel: [w828] -> w826
          tunnel: w825 -> [w828]
          tunnel: w826 -> [w852]
          frame #0 {
            n298 = call-poly <vilib>:"Read From XML File.vi"() -> ("error out"=w831:errorcluster, "XML Elements"=w832:string)  [unwired: 9 in, 1 out]
            n299 = Unbundle By Name(w831) -> ("status"=w829:bool)
            n300 = property on="Datenspeicher" class="Cluster (strikt)"() -> ("Value"=w827:T3)  [unwired: 2 in, 2 out]
            n301 = Not(x=w829) -> (.not. x?=w830:bool)
            n302 = case shown="True" w830 {
              tunnel: w832 -> [_ w851]
              tunnel: w827 -> [_ w850]
              frame False {
              }
              frame True {
                n303 = Unflatten From XML(xml string=w851, type=w850) -> (value=w849:T3)  [unwired: 1 in, 1 out]
                n304 = Unbundle(w849) -> ("Fahrzeugdaten"=w848:string, "Rolle [Inkr/U]"=w847:u16, "Rollenumfang [m]"=w846:dbl, "Rollenträgheit [kgm²]"=w845:dbl, "Zündung [Imp/U]"=w844:u8, "Getriebe [1:]"=w843:dbl, "Reifenumfang [m]"=w842:dbl, "Gl. Mittelwert"=w841:u8, "Differenzenquotient"=w840:u8, "Polynom"=w839:u8, "Lufttemperatur [°C]"=w838:dbl, "Luftfeuchtigkeit [%]"=w837:dbl, "Luftdruck [mbar]"=w836:dbl, "Übersetzung ermitteln aus"=w833:u8, "[s]"=w835:dbl, "n vom Gas [1/min]"=w834:dbl)  [unwired: 12 out]
                n305 = property on="Polynom" class="DigWert (strikt)"("Value"=w839) -> ()  [unwired: 2 in, 2 out]
                n306 = property on="Dauer [s]" class="DigWert (strikt)"("Value"=w835) -> ()  [unwired: 2 in, 2 out]
                n307 = property on="Fahrzeugdaten" class="Str"("Value"=w848) -> ()  [unwired: 2 in, 2 out]
                n308 = property on="Rolle [Inkr/U]" class="DigWert (strikt)"("Value"=w847) -> ()  [unwired: 2 in, 2 out]
                n309 = property on="Rollenumfang [m]" class="DigWert (strikt)"("Value"=w846) -> ()  [unwired: 2 in, 2 out]
                n310 = property on="Rollenträgheit [kgm²]" class="DigWert (strikt)"("Value"=w845) -> ()  [unwired: 2 in, 2 out]
                n311 = property on="Zündung [Imp/U]" class="DigWert (strikt)"("Value"=w844) -> ()  [unwired: 2 in, 2 out]
                n312 = property on="Getriebe [1:]" class="DigWert (strikt)"("Value"=w843) -> ()  [unwired: 2 in, 2 out]
                n313 = property on="Reifenumfang [m]" class="DigWert (strikt)"("Value"=w842) -> ()  [unwired: 2 in, 2 out]
                n314 = property on="Gleitender Mittelwert" class="DigWert (strikt)"("Value"=w841) -> ()  [unwired: 2 in, 2 out]
                n315 = property on="Differenzenquotient" class="DigWert (strikt)"("Value"=w840) -> ()  [unwired: 2 in, 2 out]
                n316 = property on="Lufttemperatur [°C]" class="DigWert (strikt)"("Value"=w838) -> ()  [unwired: 2 in, 2 out]
                n317 = property on="Luftfeuchtigkeit [%]" class="DigWert (strikt)"("Value"=w837) -> ()  [unwired: 2 in, 2 out]
                n318 = property on="Luftdruck [mbar]" class="DigWert (strikt)"("Value"=w836) -> ()  [unwired: 2 in, 2 out]
                n319 = property on="Übersetzung ermitteln aus" class="Enum (strikt)"("Value"=w833) -> ()  [unwired: 2 in, 2 out]
                n320 = property on="n vom Gas [1/min]" class="DigWert (strikt)"("Value"=w834) -> ()  [unwired: 2 in, 2 out]
              }
            }
          }
          frame #1 {
            n321 = property on="Konfiguration:" class="Bool. (strikt)"("Value"=w852) -> ()  [unwired: 2 in, 2 out]
          }
        }
      }
      event "Drucken": Value Change {
        n322 = event-data() -> ("OldVal"=w853:bool)  [unwired: 1 in, 5 out]
        n323 = flat-sequence {
          tunnel: [w855] -> w854
          tunnel: w853 -> [w855]
          tunnel: w854 -> [w872]
          frame #0 {
            n324 = control-ref of="XY-Graph"() -> (w863:refnum<vi>)
            n325 = call <vilib>:"New Report.vi"("report type"=enum16{"Standard Report", "HTML"}."Standard Report") -> ("report out"=w858:refnum<class "NI_report.lvclass">, "error out"=w859:errorcluster)  [unwired: 13 in]
            n326 = property on="Fahrzeugdaten" class="Str"() -> ("Value"=w857:string)  [unwired: 2 in, 2 out]
            n327 = call-dynamic "Append Control Image to Report.vi"("report in"=w858, "image depth"=24, "ctrl reference"=w863, "error in (no error)"=w859) -> ("report out"=w865:refnum<class "NI_report.lvclass">, "error out"=w864:errorcluster)  [unwired: 8 in, 2 out]
            n328 = call-poly <vilib>:"Append Report Text.vi"("report in"=w865, "text"=w857, "error in (no error)"=w864) -> ("report out"=w866:refnum<class "NI_report.lvclass">, "error out"=w867:errorcluster)  [unwired: 9 in, 2 out]
            n329 = property on="Ergebnis" class="Str"() -> ("Value"=w856:string)  [unwired: 2 in, 2 out]
            n330 = call-poly <vilib>:"Append Report Text.vi"("report in"=w866, "text"=w856, "append on new line? (F)"=TRUE, "error in (no error)"=w867) -> ("report out"=w868:refnum<class "NI_report.lvclass">, "error out"=w869:errorcluster)  [unwired: 8 in, 2 out]
            n331 = call-dynamic "Print Report.vi"("report in"=w868, "error in (no error)"=w869) -> ("report out"=w862:refnum<class "NI_report.lvclass">, "error out"=w861:errorcluster)  [unwired: 12 in]
            n332 = call-dynamic "Dispose Report.vi"("report in"=w862, "error in (no error)"=w861) -> ()  [unwired: 13 in, 1 out]
          }
          frame #1 {
            n333 = property on="Drucken" class="Bool. (strikt)"("Value"=w872) -> ()  [unwired: 2 in, 2 out]
          }
        }
      }
      event "Speichern": Value Change {
        n334 = event-data() -> ("OldVal"=w873:bool)  [unwired: 1 in, 5 out]
        n335 = local read "Datenspeicher"() -> (w874:T3)
        n336 = local write "Speichern"(w873) -> ()
        n337 = Flatten To XML(anything=w874) -> (xml string=w876:string)
        n338 = call-poly <vilib>:"Write to XML File.vi"("XML Input"=w876) -> ("error out"=w875:errorcluster)  [unwired: 8 in, 2 out]
        n339 = case shown="Kein Fehler" w875 {
          frame No Error {
          }
          frame Error {
          }
        }
      }
      event "Ende": Value Change {
        n340 = event-data() -> ("OldVal"=w877:bool)  [unwired: 1 in, 5 out]
        n341 = local write "Ende"(w877) -> ()
      }
      event "Serielle Schnittstelle": Value Change {
        n342 = event-data() -> ()  [unwired: 1 in, 6 out]
        n343 = property on="Start [F1]" class="Bool. (strikt)"("DisabledEnum"=T5."Enabled" ("Deaktiviert")) -> ()  [unwired: 2 in, 2 out]
      }
      event "Messung": Value Change {
        n344 = event-data() -> ("NewVal"=w880:bool)  [unwired: 1 in, 5 out]
        n345 = case shown="True" w880 {
          frame True {
            w881 = T5."Disabled and Grayed Out" ("Deaktiviert")
            n346 = property on="Lufttemperatur [°C]" class="DigWert (strikt)"("DisabledEnum"=w881) -> ()  [unwired: 2 in, 2 out]
            n347 = property on="Luftdruck [mbar]" class="DigWert (strikt)"("DisabledEnum"=w881) -> ()  [unwired: 2 in, 2 out]
            n348 = property on="Luftfeuchtigkeit [%]" class="DigWert (strikt)"("DisabledEnum"=w881) -> ()  [unwired: 2 in, 2 out]
          }
          frame False {
            w882 = T5."Enabled" ("Deaktiviert")
            n349 = property on="Lufttemperatur [°C]" class="DigWert (strikt)"("DisabledEnum"=w882) -> ()  [unwired: 2 in, 2 out]
            n350 = property on="Luftdruck [mbar]" class="DigWert (strikt)"("DisabledEnum"=w882) -> ()  [unwired: 2 in, 2 out]
            n351 = property on="Luftfeuchtigkeit [%]" class="DigWert (strikt)"("DisabledEnum"=w882) -> ()  [unwired: 2 in, 2 out]
          }
        }
      }
      event "Übersetzung ermitteln aus": Value Change {
        n352 = event-data() -> ("NewVal"=w883:T2)  [unwired: 1 in, 5 out]
        n353 = case shown="\"nKuWe / nRolle\"" w883 {
          tunnel: [T5."Disabled and Grayed Out" ("Deaktiviert") T5."Disabled and Grayed Out" ("Deaktiviert") T5."Enabled" ("Deaktiviert")] -> w886
          frame "nKuWe / nRolle" {
          }
          frame "Zündsignal", Default {
          }
          frame "Getriebe & Reifen" {
          }
        }
        n354 = case shown="\"Zündsignal\", Standard" w883 {
          tunnel: [T5."Enabled" ("Deaktiviert") T5."Disabled and Grayed Out" ("Deaktiviert") T5."Disabled and Grayed Out" ("Deaktiviert")] -> w884
          frame "nKuWe / nRolle" {
          }
          frame "Zündsignal", Default {
          }
          frame "Getriebe & Reifen" {
          }
        }
        n355 = case shown="\"Zündsignal\", Standard" w883 {
          tunnel: [T5."Disabled and Grayed Out" ("Deaktiviert") T5."Enabled" ("Deaktiviert") T5."Disabled and Grayed Out" ("Deaktiviert")] -> w885
          frame "nKuWe / nRolle" {
          }
          frame "Zündsignal", Default {
          }
          frame "Getriebe & Reifen" {
          }
        }
        n356 = property on="Getriebe [1:]" class="DigWert (strikt)"("DisabledEnum"=w886) -> ()  [unwired: 2 in, 2 out]
        n357 = property on="Reifenumfang [m]" class="DigWert (strikt)"("DisabledEnum"=w886) -> ()  [unwired: 2 in, 2 out]
        n358 = property on="nKuWe/nRolle" class="DigWert (strikt)"("DisabledEnum"=w884) -> ()  [unwired: 2 in, 2 out]
        n359 = property on="Zündung [Imp/U]" class="DigWert (strikt)"("DisabledEnum"=w885) -> ()  [unwired: 2 in, 2 out]
      }
    }
  }
